vi "Stereo - Calibrate Single Camera.vi"(8 "error in (no error)":errorcluster, 10 "Calibration Grids":T4(array[cluster]), 11 "Image in":T1) -> (0 "error out":errorcluster, 2 "Insufficient Data":bool, 3 "Image out":T1)   [LabVIEW 2014]
doc: "Learns the camera model for a single camera."
uses:
  <vilib>/vision/Image Controls.llb/IMAQ Image.ctl
  <vilib>/vision/Calibration.llb/Calibration Reference Points.ctl
  <vilib>/vision/Image Controls.llb/Vision Info Type2.ctl
  <vilib>/vision/NI_Vision_Development_Module.lvlib
panel:
  # "Overview: Learns the camera model for a single camera."
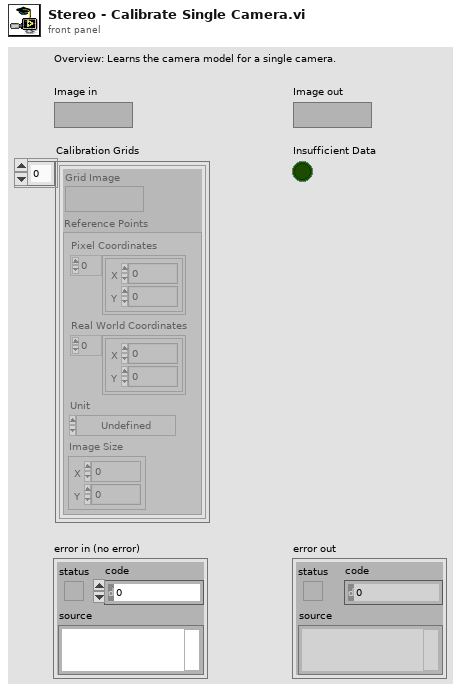
[diagram p1: front panel]
types:
  T1 = typedef "IMAQ Image.ctl" = refnum<image>
  T2 = typedef "Calibration Reference Points.ctl" = cluster{"Pixel Coordinates":cluster{"X":dbl, "Y":dbl}[], "Real World Coordinates":cluster{"X":dbl, "Y":dbl}[], "Unit":T3, "Image Size":cluster{"X":u32, "Y":u32}}
  T3 = typedef "Image Unit" = enum32{"Undefined", "Angström", "Micrometer", "Millimeter", "Centimeter", "Meter", "Kilometer", "Microinch", "Inch", "Feet", "Nautical miles", "Standard miles", "Steps"}
  T4 = cluster{"Grid Image":T1, "Reference Points":T2}[]
  T5 = typedef "Vision Info Type2.ctl" = u32
  T6 = typedef "Internal Parameters.ctl" = cluster{"Insufficient Data":bool, "Focal Length (pixel)":cluster{"fx":sgl, "fy":sgl}, "Optical Center (pixel)":cluster{"cx":sgl, "cy":sgl}}
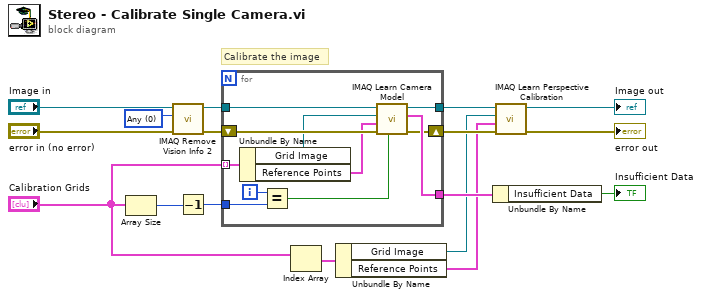
[diagram p0: block diagram]
diagram:
  w15 = T5 0 items=["Any", "Calibration", "Overlay", "Grayscale Template", "Color Template", "Geometric Template", "Custom Data", "Golden Template", "Geometric Template 2", "Contour Data", "Camera Model"] ("Vision Info")
  # "Calibrate the image"
  n1 = Array Size(array="Calibration Grids") -> (size(s)=w17:i32)
  n2 = call "IMAQ Remove Vision Info 2"("error in (no error)"="error in (no error)", "Vision Info"=w15, "Image"="Image in") -> ("error out"=w12:errorcluster, "Image Out"=w13:T1)  [unwired: 7 out]
  n3 = Decrement(x=w17) -> (x-1=w14:i32)
  n4 = for {
    tunnel: w14 -> [w27]
    tunnel: [w25] -> w16
    tunnel: w13 -> [w24]
    tunnel: "Calibration Grids" -> [w20] mode=indexing
    tunnel: [w19] -> w8
    shift-right: [w23] -> w6
    shift-left: w12 -> [w22]
    i -> [w28]
    n5 = Unbundle By Name(w20) -> ("Grid Image"=w18:T1, "Reference Points"=w21:T2)
    n6 = Equal?(x=w28, y=w27) -> (x = y?=w26:bool)
    n7 = call "IMAQ Learn Camera Model"("Add Points and Learn (True)"=w26, "error in (no error)"=w22, "Reference Points"=w21, "Image"=w18, "Calibration Template Image"=w24) -> ("error out"=w23:errorcluster, "Internal Parameters"=w25:T6, "Calibration Template Image Out"=w19:T1)  [unwired: 1 in, 3 out]
  }
  n8 = Index Array(array="Calibration Grids") -> (element=w4:cluster{"Grid Image":T1, "Reference Points":T2})  [unwired: 1 in]
  n9 = Unbundle By Name(w4) -> ("Grid Image"=w3:T1, "Reference Points"=w2:T2)
  n10 = Unbundle By Name(w16) -> ("Insufficient Data"=→"Insufficient Data":bool)
  n11 = call "IMAQ Learn Perspective Calibration"("error in (no error)"=w6, "Reference Points"=w2, "Image"=w3, "Calibration Template Image"=w8) -> ("error out"=→"error out":errorcluster, "Calibration Template Image Out"=→"Image out":T1)  [unwired: 6 out]
